vi "Format_Relay_out.vi"(10 "Set_Channel_Relay":T1 {"Relay_CH_Array"."OUTPUT_Relay_Channels" items=["CONN_SUPPLY_%d_FCT", "HB_CONN_%d_FCT", "L_IND_CONN_%d_FCT", "R_IND_CONN_%d_FCT", "SW1_%d_FCT", "SW2_%d_FCT", "CAN_H_%d_FCT", "CAN_L_%d_FCT", "CYLINDER_ON/OFF_%d_FCT", "SPARE_1_%d_FCT", "SPARE_2_%d_FCT", "Tower Red", "Tower Amber", "Tower Green", "Tower Buzzer", "SLIMRELAY_DUT_%d_FCT", "GND_DMM_%d_EOL", "CAN_H_RES_%d_EOL", "CAN_L_RES_%d_EOL", "L_IND_RES_%d_EOL", "R_IND_RES_%d_EOL", "HB_CONN_DMM_%d_EOL", "14V_RES_%d_EOL", "CAN_L_(DMM-)_%d_EOL", "CAN_H_%d_EOL", "CAN_L_%d_EOL", "14V_%d_EOL", "GND_%d_EOL", "HB_CONN_%d_EOL", "L_IND_%d_EOL", "R_IND_%d_EOL", "CYLINDER_DUT_%d_EOL", "CYL_PB_1_%d_EOL", "CYL_PB_2_%d_EOL", "DUT_PASS_%d_EOL", "DUT_FAIL_%d_EOL", "SPARE1_%d_EOL", "Tower Red_EOL", "Tower Amber_EOL", "Tower Green_EOL", "Tower Buzzer_EOL"]}, 11 "DUT":string) -> (1 "Array":T3[](array[typedef]), 2 "output cluster":T1 {"Relay_CH_Array"."OUTPUT_Relay_Channels" items=["CONN_SUPPLY_%d_FCT", "HB_CONN_%d_FCT", "L_IND_CONN_%d_FCT", "R_IND_CONN_%d_FCT", "SW1_%d_FCT", "SW2_%d_FCT", "CAN_H_%d_FCT", "CAN_L_%d_FCT", "CYLINDER_ON/OFF_%d_FCT", "SPARE_1_%d_FCT", "SPARE_2_%d_FCT", "Tower Red", "Tower Amber", "Tower Green", "Tower Buzzer", "SLIMRELAY_DUT_%d_FCT", "GND_DMM_%d_EOL", "CAN_H_RES_%d_EOL", "CAN_L_RES_%d_EOL", "L_IND_RES_%d_EOL", "R_IND_RES_%d_EOL", "HB_CONN_DMM_%d_EOL", "14V_RES_%d_EOL", "CAN_L_(DMM-)_%d_EOL", "CAN_H_%d_EOL", "CAN_L_%d_EOL", "14V_%d_EOL", "GND_%d_EOL", "HB_CONN_%d_EOL", "L_IND_%d_EOL", "R_IND_%d_EOL", "CYLINDER_DUT_%d_EOL", "CYL_PB_1_%d_EOL", "CYL_PB_2_%d_EOL", "DUT_PASS_%d_EOL", "DUT_FAIL_%d_EOL", "SPARE1_%d_EOL", "Tower Red_EOL", "Tower Amber_EOL", "Tower Green_EOL", "Tower Buzzer_EOL"]}, 3 "OUTPUT_Relay_Channels":T2 items=["CONN_SUPPLY_%d_FCT", "HB_CONN_%d_FCT", "L_IND_CONN_%d_FCT", "R_IND_CONN_%d_FCT", "SW1_%d_FCT", "SW2_%d_FCT", "CAN_H_%d_FCT", "CAN_L_%d_FCT", "CYLINDER_ON/OFF_%d_FCT", "SPARE_1_%d_FCT", "SPARE_2_%d_FCT", "Tower Red", "Tower Amber", "Tower Green", "Tower Buzzer", "SLIMRELAY_DUT_%d_FCT", "GND_DMM_%d_EOL", "CAN_H_RES_%d_EOL", "CAN_L_RES_%d_EOL", "L_IND_RES_%d_EOL", "R_IND_RES_%d_EOL", "HB_CONN_DMM_%d_EOL", "14V_RES_%d_EOL", "CAN_L_(DMM-)_%d_EOL", "CAN_H_%d_EOL", "CAN_L_%d_EOL", "14V_%d_EOL", "GND_%d_EOL", "HB_CONN_%d_EOL", "L_IND_%d_EOL", "R_IND_%d_EOL", "CYLINDER_DUT_%d_EOL", "CYL_PB_1_%d_EOL", "CYL_PB_2_%d_EOL", "DUT_PASS_%d_EOL", "DUT_FAIL_%d_EOL", "SPARE1_%d_EOL", "Tower Red_EOL", "Tower Amber_EOL", "Tower Green_EOL", "Tower Buzzer_EOL"])   [LabVIEW 2024, in "Launcher_DTU.lvlib"]
uses:
  Launcher_DTU.lvlib
  Modules/Relay_Module/support/Relay_Enum_OUT.ctl
  Modules/Relay_Module/Relay_Module.lvlib
  Modules/Settings/support/Common_plc_DOs.ctl
  Modules/Settings/Setting_Screen.lvlib
  Modules/Settings/support/Relay_Channel_Array.ctl
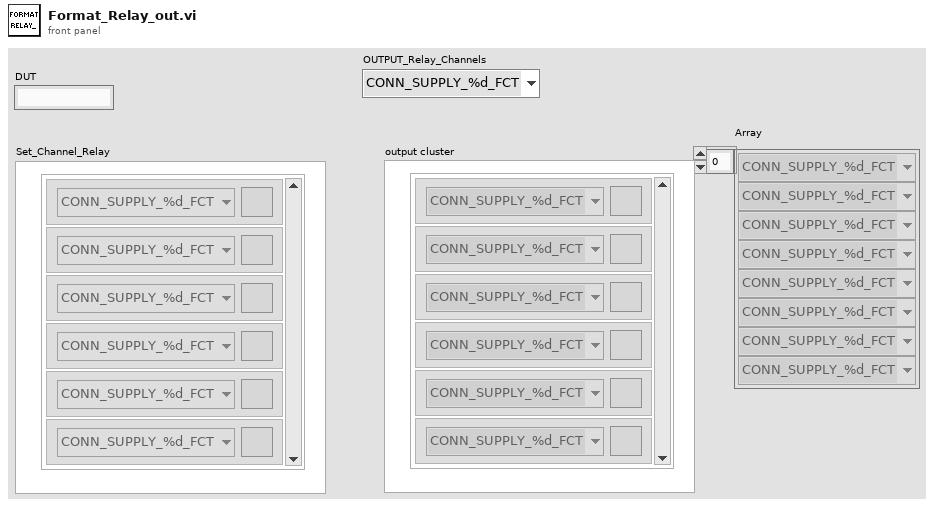
[diagram p1: front panel]
types:
  T1 = typedef "Setting_Screen.lvlib/Relay_Channel_Array.ctl" = cluster{"Relay_CH_Array":cluster{"OUTPUT_Relay_Channels":T2, "On/Off":bool}[]}
  T2 = typedef "Setting_Screen.lvlib/Common_plc_DOs.ctl" = u16
  T3 = typedef "Relay_Module.lvlib/Relay_Enum_OUT.ctl" = enum16{"CONN_SUPPLY_%d_FCT", "HB_CONN_%d_FCT", "L_IND_CONN_%d_FCT", "R_IND_CONN_%d_FCT", "SW1_%d_FCT", "SW2_%d_FCT", "CAN_H_%d_FCT", "CAN_L_%d_FCT", "CYLINDER_ON/OFF_%d_FCT", "SPARE_1_%d_FCT", "SPARE_2_%d_FCT", "Tower Red", "Tower Amber", "Tower Green", "Tower Buzzer", "SLIMRELAY_DUT_%d_FCT", "GND_DMM_%d_EOL", "CAN_H_RES_%d_EOL", "CAN_L_RES_%d_EOL", "L_IND_RES_%d_EOL", "R_IND_RES_%d_EOL", "HB_CONN_DMM_%d_EOL", "14V_RES_%d_EOL", "CAN_L_(DMM-)_%d_EOL", "CAN_H_%d_EOL", "CAN_L_%d_EOL", "14V_%d_EOL", "GND_%d_EOL", "HB_CONN_%d_EOL", "L_IND_%d_EOL", "R_IND_%d_EOL", "CYLINDER_DUT_%d_EOL", "CYL_PB_1_%d_EOL", "CYL_PB_2_%d_EOL", "DUT_PASS_%d_EOL", "DUT_FAIL_%d_EOL", "SPARE1_%d_EOL", "Tower Red_EOL", "Tower Amber_EOL", "Tower Green_EOL", "Tower Buzzer_EOL"}
  T4 = cluster{"OUTPUT_Relay_Channels":T2, "On/Off":bool}[]
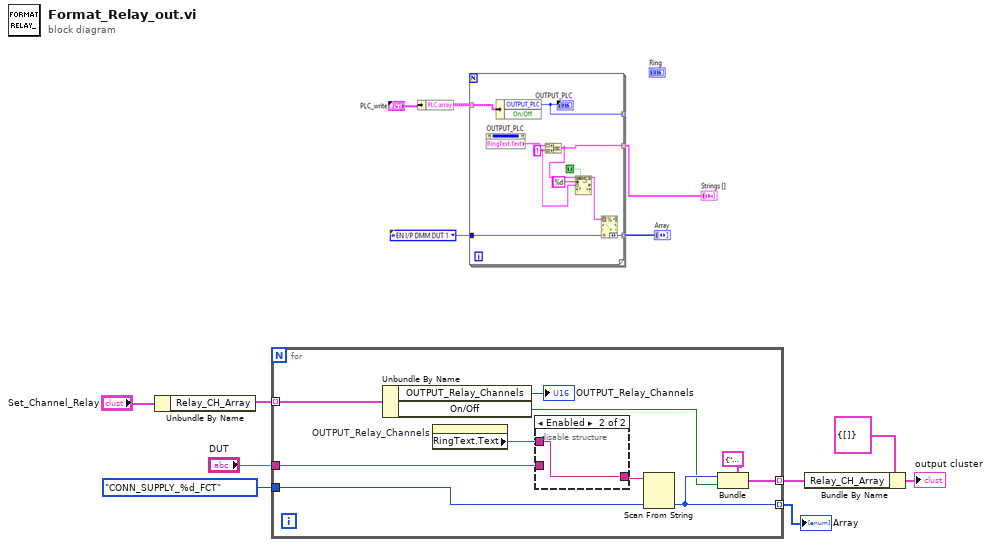
[diagram p0: block diagram]
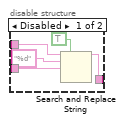
[diagram p2: hidden frame]
diagram:
  n1 = Unbundle By Name("Set_Channel_Relay") -> ("Relay_CH_Array"=w8:T4)
  n2 = for {
    tunnel: w8 -> [w11] mode=indexing
    tunnel: Relay_Enum_OUT."CONN_SUPPLY_%d_FCT" ("OUTPUT_CH_Relay") -> [w17]
    tunnel: "DUT" -> [w16]
    tunnel: [w15] -> w4 mode=indexing
    tunnel: [w13] -> w2 mode=indexing
    n3 = Unbundle By Name(w11) -> ("OUTPUT_Relay_Channels"=→"OUTPUT_Relay_Channels":T2, "On/Off"=w14:bool)
    n4 = property on="OUTPUT_Relay_Channels" class="Ring (strict)"() -> ("RingText.Text"=w9:string)  [unwired: 2 in, 2 out]
    n5 = disable-structure shown="Enabled" {
      disable-tunnel: [w21 w24] -> w18
      disable-tunnel: w16 -> [w20 _]
      disable-tunnel: w9 -> [w19 w24]
      frame Disabled {
        n6 = Search and Replace String(replace all?=TRUE ("replace all? (F)"), input string=w19, search string="%d", replace string=w20) -> (result string=w21:string)  [unwired: 4 in, 3 out]
      }
      frame Enabled {
      }
    }
    n7 = Scan From String(input string=w18, default 1=w17) -> (output 1=w15:T3)  [unwired: 3 in, 3 out]
    n8 = Bundle(cluster=cluster{"OUTPUT_CH_Relay":T3, "On/Off":bool} {"OUTPUT_CH_Relay"=enum."CONN_SUPPLY_%d_FCT", "On/Off"=FALSE}, "OUTPUT_CH_Relay"=w15, "On/Off"=w14) -> (w13:cluster{"OUTPUT_CH_Relay":T3, "On/Off":bool})
  }
  "Array" <- w4
  n9 = Bundle By Name(cluster=T1 {"Relay_CH_Array"=[]} ("Set_Channel_Relay"), "Relay_CH_Array"=w2) -> (→"output cluster":T1)
